vi "Get Data.vi"(8 "error in (no error)":errorcluster, 10 "index":i32, 11 "Impulse Manager in":refnum<class "Impulse Manager.lvclass">) -> (0 "error out":errorcluster, 2 "Data out":dbl[][](array[numeric]), 3 "Impulse Manager out":refnum<class "Impulse Manager.lvclass">)   [LabVIEW 2016, in "Impulse Manager.lvclass"]
uses:
  Impulse Manager.lvclass
  Impulse Manager.lvclass/Impulse Manager.ctl
  Desaccade Manipulator/Desaccade Manipulator.lvclass
  Impulse Data/Impulse Data.lvclass
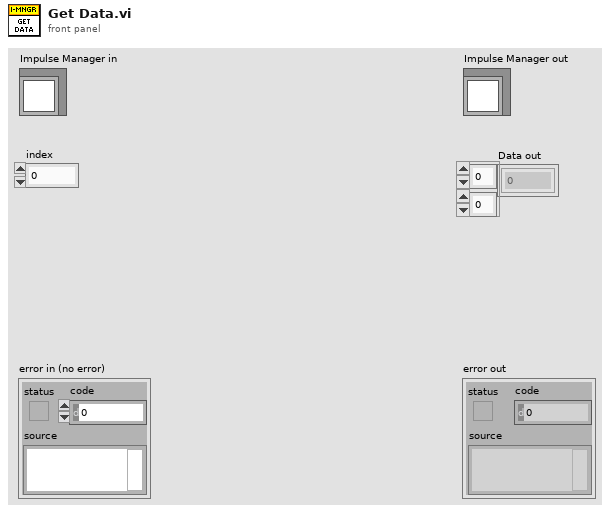
[diagram p1: front panel]
types:
  T1 = typedef "Impulse Data.lvclass/Instance handle.ctl" = refnum<data-value>
  T2 = typedef "core.lvlib/TD_Impulse Parameter.ctl" = cluster{"Color":u32, "Visible":bool, "Channel":u16, "Invert":bool, "Desaccade":bool, "Offset":dbl, "Gain":dbl}[]
  T3 = cluster{"Color":u32, "Visible":bool, "Channel":u16, "Invert":bool, "Desaccade":bool, "Offset":dbl, "Gain":dbl}
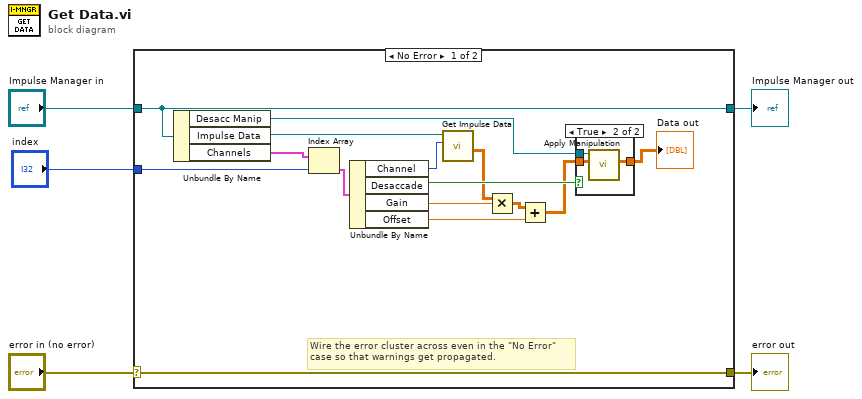
[diagram p0: block diagram]
diagram:
  n1 = case shown="No Error" "error in (no error)" {
    selector: "error in (no error)" -> [w20 w26]
    tunnel: [w20 w26] -> w4
    tunnel: [w19 w25] -> w2
    tunnel: "Impulse Manager in" -> [w19 w25]
    tunnel: "index" -> [w17 _]
    frame No Error {
      # "Wire the error cluster across even in the \"No Error\"\ncase so that warnings get propagated."
      n2 = Unbundle By Name(w19) -> ("Desacc Manip"=w13:refnum<class "Desaccade Manipulator.lvclass">, "Impulse Data"=w16:T1, "Channels"=w18:T2)
      n3 = Index Array(array=w18, index=w17) -> (element=w15:T3)
      n4 = Unbundle By Name(w15) -> ("Channel"=w14:u16, "Desaccade"=w11:bool, "Gain"=w9:dbl, "Offset"=w7:dbl)
      n5 = call "Get Impulse Data.vi"("Channel"=w14, "Reference in"=w16) -> ("Impulses out"=w10:dbl[][])  [unwired: 8 in, 1 out]
      n6 = Multiply(x=w10, y=w9) -> (x*y=w8:dbl[][])
      n7 = Add(x=w8, y=w7) -> (x+y=w6:dbl[][])
      n8 = case shown="True" w11 {
        tunnel: w6 -> [w21 w24]
        tunnel: [w21 w23] -> w12
        tunnel: w13 -> [_ w22]
        frame False {
        }
        frame True {
          n9 = call-dynamic "Apply Manipulation.vi"("Data in"=w24, "Desaccade Manipulator in"=w22) -> ("Data out"=w23:dbl[][])  [unwired: 7 in, 2 out]
        }
      }
      "Data out" <- w12
    }
    frame Error {
    }
  }
  "error out" <- w4
  "Impulse Manager out" <- w2
